vi "GOOP_MyComputer_Item_Exit.vi"(11 "Object":u64) -> ()   [LabVIEW 2014]
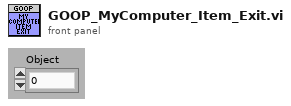
[diagram p1: front panel]
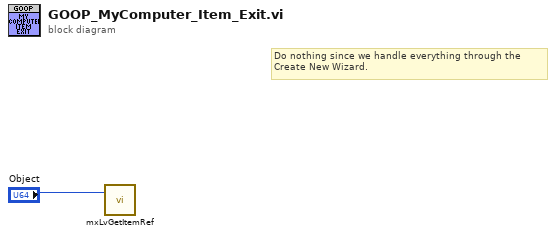
[diagram p0: block diagram]
diagram:
  # "Do nothing since we handle everything through the\nCreate New Wizard."
  n1 = call <resource>:"mxLvGetItemRef.vi"("Item"="Object") -> ()  [unwired: 1 in, 3 out]
